vi "Initialize.vi"(8 "error in (no error)":errorcluster) -> (0 "error out":errorcluster)   [LabVIEW 2018, in "Tag Engine.lvlib" / "Tag Core.lvclass"]
doc: "Initialize the Tag store.\n\nCall this VI at the startup of your main process (that does not leave memory until your application is stopped). The Tag store will be owned by this process."
uses:
  Tag Core.lvclass
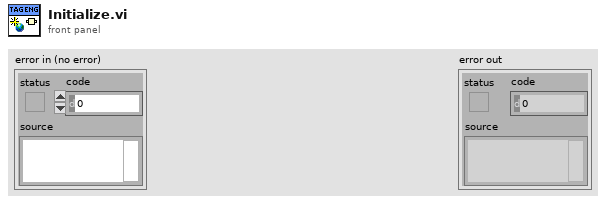
[diagram p1: front panel]
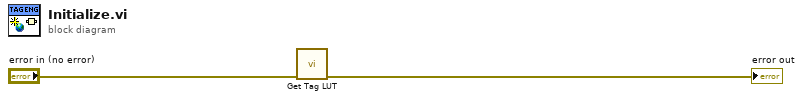
[diagram p0: block diagram]
diagram:
  n1 = call "Get Tag LUT.vi"("error in (no error)"="error in (no error)") -> ("error out"=→"error out":errorcluster)  [unwired: 9 in, 1 out]
